vi "Find_Slave_Data.vi"(4 "Process data parameters in":T2={"Stop loop"={"Settings changed?"=FALSE, "Stop?"=refnum}, "Button refs"={"Stop program"=refnum, "Save settings"=refnum, "DAQ mode"=refnum, "Reset settings"=refnum, "Apply settings"=refnum, "Reset MAS"=refnum, "Reset SLV"=refnum, "Local DBase?"=refnum, "Last value DBase"=FALSE, "Database"=refnum, "Calibration"=refnum, "Save settings 2"=refnum}, "Process messages"={"Process message mode"=enum."Error", "Slave data?"=FALSE, "Length get settings message"=0, "Delta time"=0.0, "Data_Filter"={"Filter_Data"=FALSE, "Use_Thresh"=FALSE, "Reduce data?"=FALSE}, "Time_difference_stack"=[], "Starting sec"=0, "Ending sec"=0, "Ending sec 2"=0, "MAS_Page_Thresh"=refnum, "SLV_Page_Thresh"=refnum, "Database"=refnum}, "Settings state"={"MAS locked?"=refnum, "SLV locked?"=refnum}, "Mode"={"Mode"=enum."Dialog", "Expert?"=FALSE, "Dialog?"=FALSE}, "Alignment parameters"=refnum, "Timer parameters"=refnum, "Files"={"Path config file"=path "", "Path def. ini file"=path "", "Path ini file 1"=path "", "Path ini file 2"=path "", "Path RBF file"=path ""}, "Time difference"=refnum, "Alignment"={"GEN_Page_Calibrate"=refnum, "MAS_Page_Gain"=refnum, "MAS_Page_Offset"=refnum, "SLV_Page_Gain"=refnum, "SLV_Page_Offset"=refnum, "MAS_Page_Common"=refnum, "SLV_Page_Common"=refnum}, "Page Statistics"=refnum}, 6 "Queues":T11, 7 "One Second in":T12[](array[typedef]) {"Ch1 High" format="%0.0f"}, 8 "Status/Errors in":refnum<vi>, 9 "Time master":dbl, 10 "GPS timestamp master":T13, 11 "Devices":T14) -> (0 "Status/Errors out":refnum<vi>, 1 "Time delta slave":dbl, 2 "Slave data":u8[](array[numeric]), 3 "Found SLV data?":T1, 5 "One Second out":T12[](array[typedef]) {"Ch1 High" format="%0.0f"})   [LabVIEW 2010]
uses:
  Controls/Devices.ctl
  Controls/GPS_Timestamp.ctl
  Controls/One_Second.ctl
  Controls/Queues.ctl
  Controls/Process_Data_Parameters.ctl
  Controls/Stop_Loop.ctl
  Controls/Button_Refs.ctl
  Controls/Process_Messages.ctl
  Controls/Process_Message_Mode.ctl
  Controls/Settings_State.ctl
  Controls/Mode.ctl
  Controls/Files.ctl
  Controls/Page_Calibration.ctl
  Controls/Found_SLV_Data.ctl
  Controls/Comparison_Result.ctl
  Controls/Master.ctl
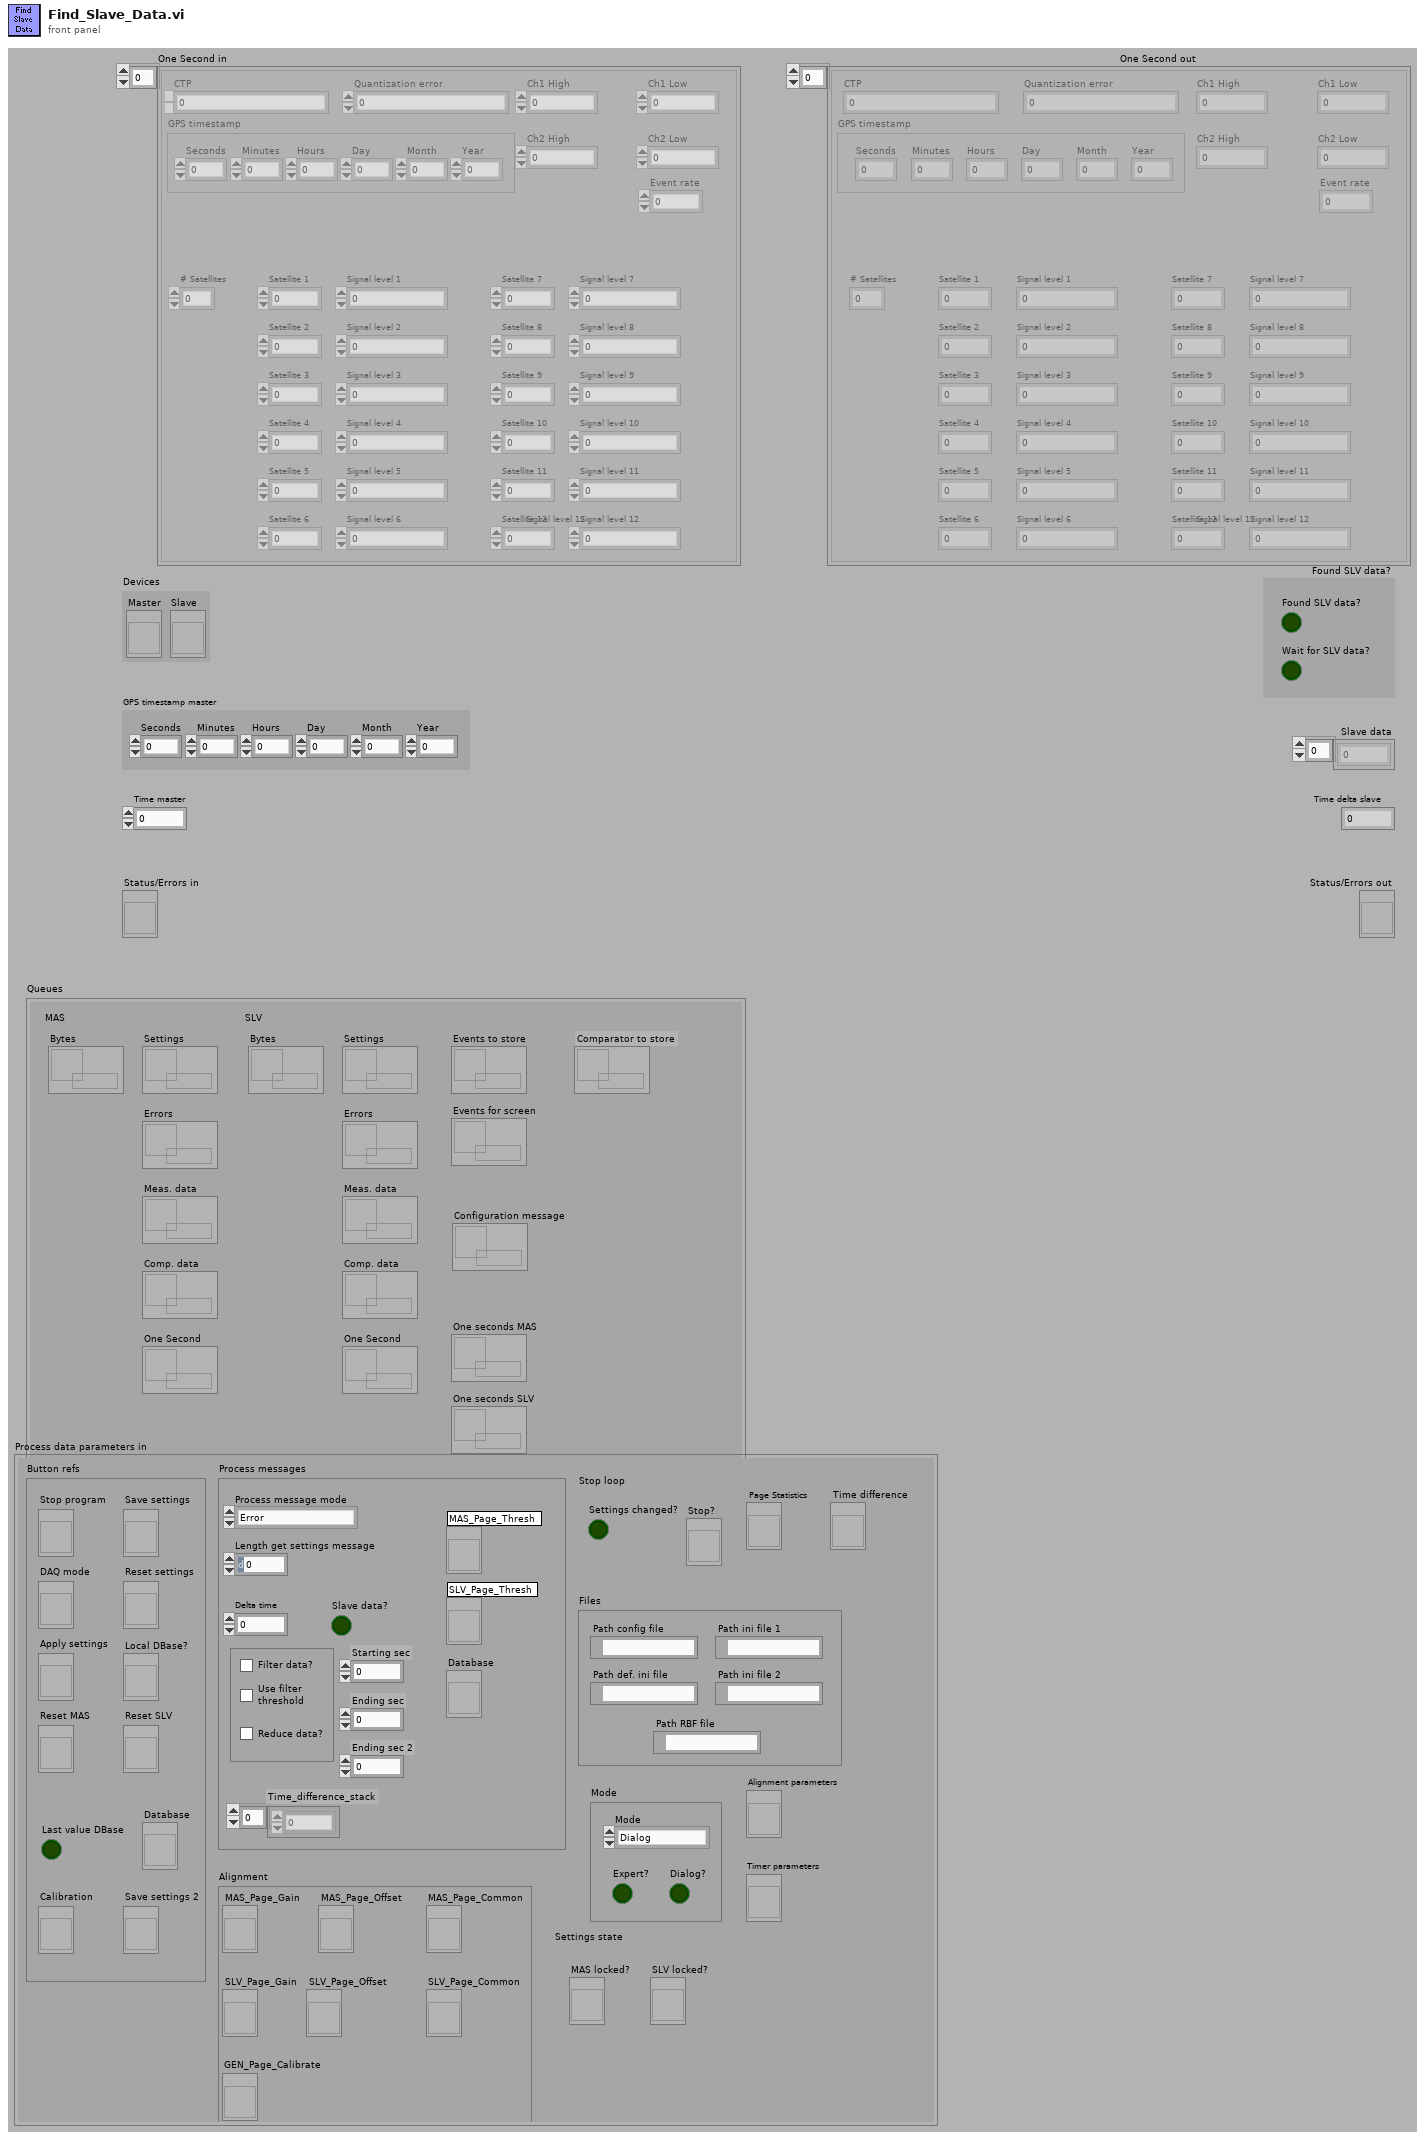
[diagram p1: front panel]
types:
  T1 = typedef "Found_SLV_Data.ctl" = cluster{"Found SLV data?":bool, "Wait for SLV data?":bool}
  T2 = typedef "Process_Data_Parameters.ctl" = cluster{"Stop loop":T3, "Button refs":T4, "Process messages":T5, "Settings state":T7, "Mode":T8, "Alignment parameters":refnum<vi>, "Timer parameters":refnum<vi>, "Files":T9, "Time difference":refnum<vi>, "Alignment":T10, "Page Statistics":refnum<vi>}
  T3 = typedef "Stop_Loop.ctl" = cluster{"Settings changed?":bool, "Stop?":refnum<vi>}
  T4 = typedef "Button_Refs.ctl" = cluster{"Stop program":refnum<vi>, "Save settings":refnum<vi>, "DAQ mode":refnum<vi>, "Reset settings":refnum<vi>, "Apply settings":refnum<vi>, "Reset MAS":refnum<vi>, "Reset SLV":refnum<vi>, "Local DBase?":refnum<vi>, "Last value DBase":bool, "Database":refnum<vi>, "Calibration":refnum<vi>, "Save settings 2":refnum<vi>}
  T5 = typedef "Process_Messages.ctl" = cluster{"Process message mode":T6, "Slave data?":bool, "Length get settings message":i32, "Delta time":dbl, "Data_Filter":cluster{"Filter_Data":bool, "Use_Thresh":bool, "Reduce data?":bool}, "Time_difference_stack":u64[], "Starting sec":u64, "Ending sec":u64, "Ending sec 2":u64, "MAS_Page_Thresh":refnum<vi>, "SLV_Page_Thresh":refnum<vi>, "Database":refnum<vi>}
  T6 = typedef "Process_Message_Mode.ctl" = enum16{"Error", "Measurement data", "Comparator data", "One Second"}
  T7 = typedef "Settings_State.ctl" = cluster{"MAS locked?":refnum<vi>, "SLV locked?":refnum<vi>}
  T8 = typedef "Mode.ctl" = cluster{"Mode":enum8{"Stop", "Dialog", "Hisparc II", "Hisparc II DAQ", "Alignment"}, "Expert?":bool, "Dialog?":bool}
  T9 = typedef "Files.ctl" = cluster{"Path config file":path, "Path def. ini file":path, "Path ini file 1":path, "Path ini file 2":path, "Path RBF file":path}
  T10 = typedef "Page_Calibration.ctl" = cluster{"GEN_Page_Calibrate":refnum<vi>, "MAS_Page_Gain":refnum<vi>, "MAS_Page_Offset":refnum<vi>, "SLV_Page_Gain":refnum<vi>, "SLV_Page_Offset":refnum<vi>, "MAS_Page_Common":refnum<vi>, "SLV_Page_Common":refnum<vi>}
  T11 = typedef "Queues.ctl" = cluster{"MAS":cluster{"Bytes":refnum<queue>, "Settings":refnum<queue>, "Errors":refnum<queue>, "Meas. data":refnum<queue>, "One Second":refnum<queue>, "Comp. data":refnum<queue>}, "SLV":cluster{"Bytes":refnum<queue>, "Settings":refnum<queue>, "Errors":refnum<queue>, "Meas. data":refnum<queue>, "One Second":refnum<queue>, "Comp. data":refnum<queue>}, "Events to store":refnum<queue>, "Events for screen":refnum<queue>, "One seconds MAS":refnum<queue>, "One seconds SLV":refnum<queue>, "Configuration message":refnum<queue>, "Comparator to store":refnum<queue>}
  T12 = typedef "One_Second.ctl" = cluster{"GPS timestamp":T13, "CTP":u32, "Quantization error":u32, "Ch1 High":u16, "Ch1 Low":u16, "Ch2 High":u16, "Ch2 Low":u16, "Event rate":u16, "# Satellites":u8, "Satellite 1":u8, "Satellite 2":u8, "Satellite 3":u8, "Satellite 4":u8, "Satellite 5":u8, "Satellite 6":u8, "Signal level 1":sgl, "Signal level 2":sgl, "Signal level 3":sgl, "Signal level 4":sgl, "Signal level 5":sgl, "Signal level 6":sgl, "Satellite 7":u8, "Satellite 8":u8, "Satellite 9":u8, "Satellite 10":u8, "Satellite 11":u8, "Satellite 12":u8, "Signal level 7":sgl, "Signal level 8":sgl, "Signal level 9":sgl, "Signal level 10":sgl, "Signal level 11":sgl, "Signal level 12":sgl}
  T13 = typedef "GPS_Timestamp.ctl" = cluster{"Seconds":u8, "Minutes":u8, "Hours":u8, "Day":u8, "Month":u8, "Year":u16}
  T14 = typedef "Devices.ctl" = cluster{"Master":refnum<vi>, "Slave":refnum<vi>}
  T15 = typedef "Master.ctl" = enum16{"Master", "Slave", "General"}
  T16 = typedef "Comparison_Result.ctl" = enum16{"equal", "1 < 2", "1 > 2", "error in 1", "error in 2", "error in both"}
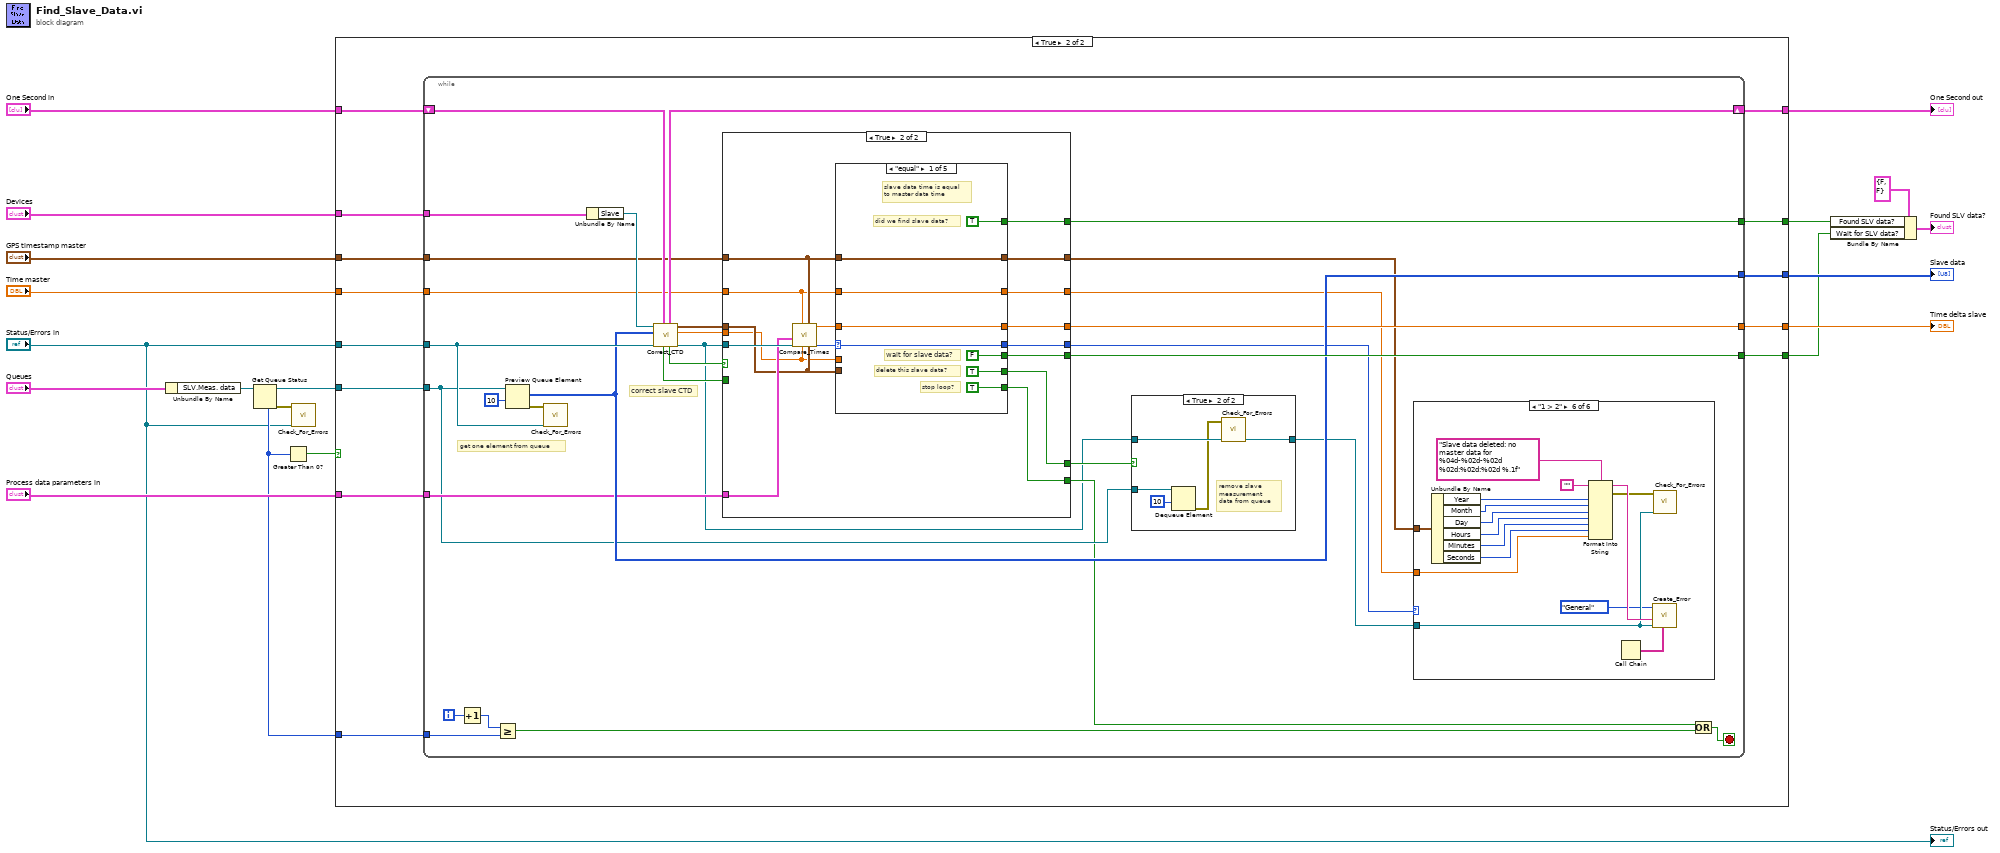
[diagram p0: block diagram]
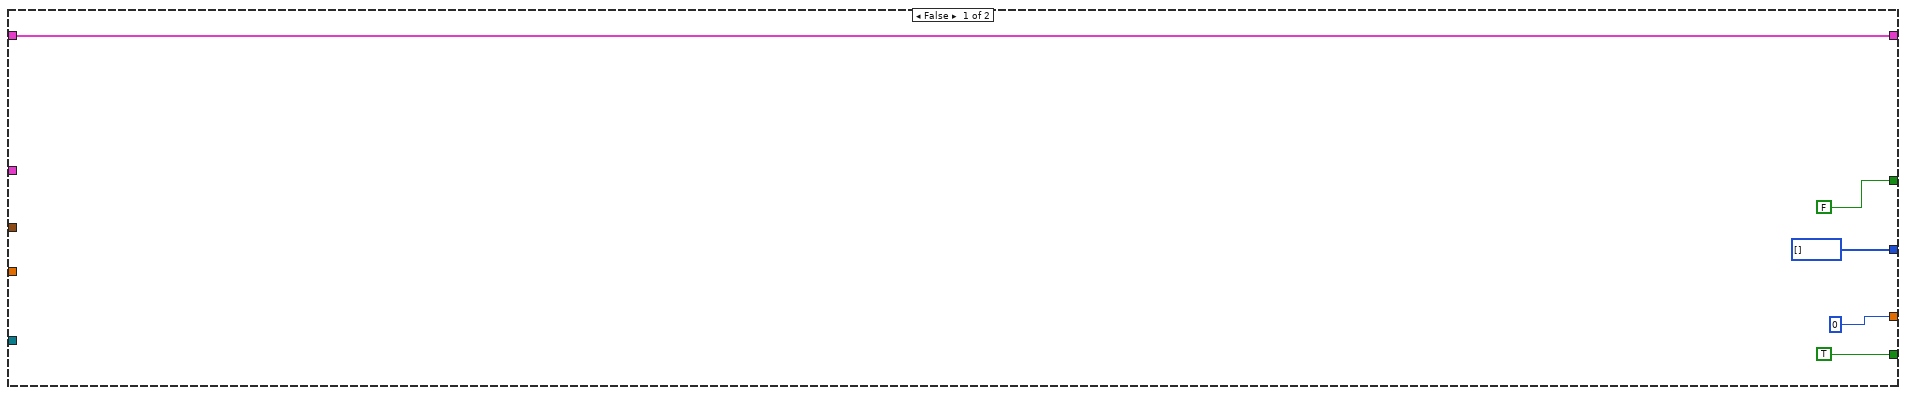
[diagram p2: hidden frame]
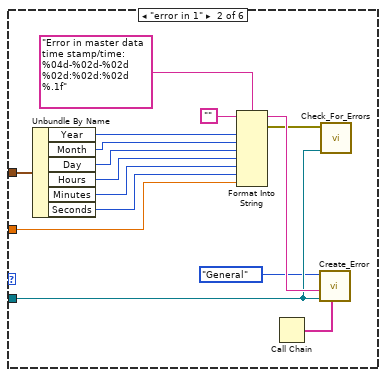
[diagram p4: hidden frame]
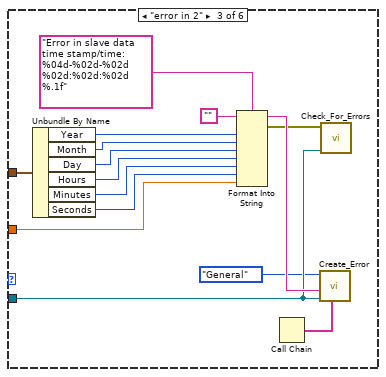
[diagram p5: hidden frame]
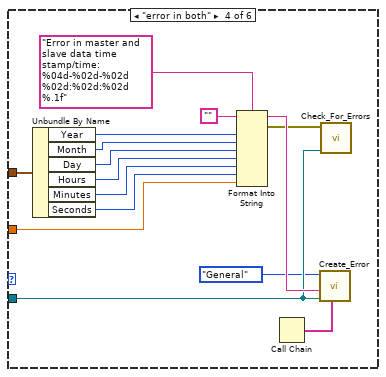
[diagram p6: hidden frame]
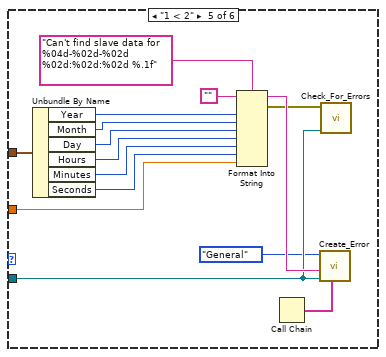
[diagram p7: hidden frame]
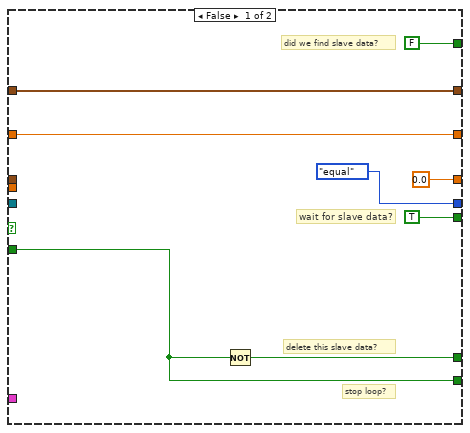
[diagram p9: hidden frame]
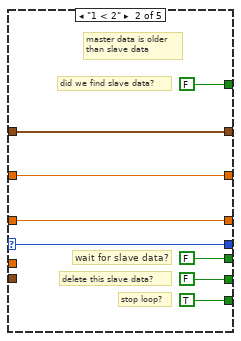
[diagram p10: hidden frame]
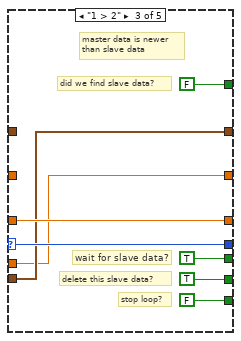
[diagram p11: hidden frame]
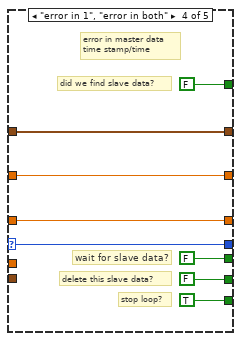
[diagram p12: hidden frame]
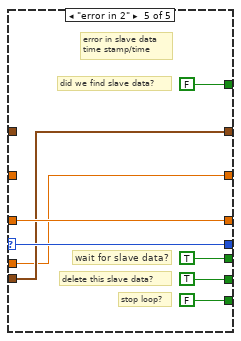
[diagram p13: hidden frame]
diagram:
  n1 = Unbundle By Name("Queues") -> ("SLV.Meas. data"=w12:refnum<queue>)
  n2 = Get Queue Status(queue=w12) -> (queue out=w11:refnum<queue>, error out=w10:errorcluster, # elements in queue=w6:i32)  [unwired: 1 in, 6 out]
  n3 = Greater Than 0?(x=w6) -> (x > 0?=w9:bool)
  n4 = call "Check_For_Errors.vi"("Status/Errors in"="Status/Errors in", "error in"=w10) -> ()  [unwired: 10 out]
  n5 = case shown="True" w9 {
    tunnel: "One Second in" -> [w22 w37]
    tunnel: [w22 w36] -> w18
    tunnel: "Status/Errors in" -> [_ w35]
    tunnel: [FALSE w30] -> w3
    tunnel: [TRUE w31] -> w2
    tunnel: "Devices" -> [_ w34]
    tunnel: "Process data parameters in" -> [_ w33]
    tunnel: "GPS timestamp master" -> [_ w26]
    tunnel: "Time master" -> [_ w25]
    tunnel: w11 -> [_ w32]
    tunnel: [u8[] [] ("Slave data") w29] -> w8
    tunnel: [0 ("CTDM slave") w28] -> w7
    tunnel: w6 -> [_ w27]
    frame False {
    }
    frame True {
      n6 = while {
        tunnel: w35 -> [w65]
        tunnel: w34 -> [w64]
        tunnel: w33 -> [w54]
        tunnel: w26 -> [w53]
        tunnel: w25 -> [w52]
        tunnel: w32 -> [w47]
        tunnel: [w58] -> w31
        tunnel: [w57] -> w30
        tunnel: [w56] -> w29
        tunnel: [w55] -> w28
        tunnel: w27 -> [w50]
        shift-right: [w62] -> w36
        shift-left: w37 -> [w63]
        i -> [w51]
        stop <- w61 stop-if-true
        # "correct slave CTD"
        # "get one element from queue"
        n7 = Increment(x=w51) -> (x+1=w49:i32)
        n8 = Greater Or Equal?(x=w49, y=w50) -> (x >= y?=w48:bool)
        n9 = Preview Queue Element(queue=w47, timeout in ms (-1)=10) -> (element=w56:u8[], error out=w67:errorcluster)  [unwired: 1 in, 2 out]
        n10 = call "Check_For_Errors.vi"("Status/Errors in"=w65, "error in"=w67) -> ()  [unwired: 10 out]
        n11 = Unbundle By Name(w64) -> ("Slave"=w66:refnum<vi>)
        n12 = call "Correct_CTD.vi"("One Second in"=w63, "Status/Errors in"=w65, "Message in"=w56, "Device in"=w66) -> ("Status/Errors out"=w42:refnum<vi>, "Time"=w43:dbl, "GPS timestamp out"=w44:T13, "CTD corrected?"=w60:bool, "One Second out"=w62:T12[], "Wait for tick count?"=w59:bool)  [unwired: 2 out]
        n13 = case shown="True" w60 {
          tunnel: w59 -> [w153 _]
          tunnel: [TRUE ("Wait for tick count?") w171] -> w58
          tunnel: [FALSE w172] -> w57
          tunnel: [0.0 ("CTDM slave") w173] -> w55
          tunnel: w54 -> [_ w166]
          tunnel: w53 -> [w151 w163]
          tunnel: w52 -> [w150 w161]
          tunnel: w44 -> [_ w160]
          tunnel: w43 -> [_ w159]
          tunnel: [w155 w170] -> w46
          tunnel: [w153 w169] -> w45
          tunnel: [Comparison_Result."equal" ("Comparison result") w168] -> w41
          tunnel: w42 -> [_ w167]
          tunnel: [w151 w164] -> w39
          tunnel: [w150 w162] -> w38
          frame False {
            # "stop loop?"
            # "delete this slave data?"
            # "wait for slave data?"
            # "did we find slave data?"
            n14 = Not(x=w153) -> (.not. x?=w155:bool)
          }
          frame True {
            n15 = call "Compare_Times.vi"("Time stamp 2"=w160, "Time stamp 1"=w163, "Time 2"=w159, "Time 1"=w161, "Status/Errors in"=w167, "Process data parameters in"=w166) -> ("Comparison result"=w165:T16, "Time 2 - 1"=w158:dbl)  [unwired: 1 in, 3 out]
            n16 = case shown="\"equal\"" w165 {
              selector: w165 -> [w176 w184 w192 w200 w208]
              tunnel: [w181 w189 w197 w205 w213] -> w173
              tunnel: w158 -> [w181 w189 w197 w205 w213]
              tunnel: [TRUE FALSE FALSE FALSE FALSE] -> w172
              tunnel: [FALSE FALSE TRUE FALSE TRUE] -> w171
              tunnel: [TRUE FALSE TRUE FALSE TRUE] -> w170
              tunnel: [TRUE TRUE FALSE TRUE FALSE] -> w169
              tunnel: [w176 w184 w192 w200 w208] -> w168
              tunnel: [w175 w183 w191 w199 w207] -> w164
              tunnel: w163 -> [w175 w183 _ w199 _]
              tunnel: [w174 w182 w190 w198 w206] -> w162
              tunnel: w161 -> [w174 w182 _ w198 _]
              tunnel: w160 -> [_ _ w191 _ w207]
              tunnel: w159 -> [_ _ w190 _ w206]
              frame "equal" {
                # "slave data time is equal\nto master data time"
                # "stop loop?"
                # "delete this slave data?"
                # "wait for slave data?"
                # "did we find slave data?"
              }
              frame "1 < 2" {
                # "master data is older\nthan slave data"
                # "stop loop?"
                # "delete this slave data?"
                # "wait for slave data?"
                # "did we find slave data?"
              }
              frame "1 > 2" {
                # "master data is newer\nthan slave data"
                # "stop loop?"
                # "delete this slave data?"
                # "wait for slave data?"
                # "did we find slave data?"
              }
              frame "error in 1", "error in both" {
                # "error in master data\ntime stamp/time"
                # "stop loop?"
                # "delete this slave data?"
                # "wait for slave data?"
                # "did we find slave data?"
              }
              frame "error in 2" {
                # "error in slave data\ntime stamp/time"
                # "stop loop?"
                # "delete this slave data?"
                # "wait for slave data?"
                # "did we find slave data?"
              }
            }
          }
        }
        n17 = case shown="True" w46 {
          tunnel: w47 -> [_ w149]
          tunnel: w42 -> [w144 w148]
          tunnel: [w144 w145] -> w40
          frame False {
            # "keep slave measurement\ndata in queue for now"
          }
          frame True {
            # "remove slave\nmeasurement\ndata from queue"
            n18 = Dequeue Element(queue=w149, timeout in ms (-1)=10) -> (error out=w147:errorcluster)  [unwired: 1 in, 3 out]
            n19 = call "Check_For_Errors.vi"("Status/Errors in"=w148, "error in"=w147) -> ("Status/Errors out"=w145:refnum<vi>)  [unwired: 9 out]
          }
        }
        n20 = case shown="\"1 > 2\"" w41 {
          tunnel: w40 -> [_ w72 w87 w102 w117 w132]
          tunnel: w39 -> [_ w82 w97 w112 w127 w142]
          tunnel: w38 -> [_ w70 w85 w100 w115 w130]
          frame Default {
          }
          frame "error in 1" {
            n21 = Unbundle By Name(w82) -> ("Year"=w79:u16, "Month"=w78:u8, "Day"=w77:u8, "Hours"=w76:u8, "Minutes"=w75:u8, "Seconds"=w74:u8)
            n22 = Format Into String(format string="Error in master data time stamp/time: %04d-%02d-%02d %02d:%02d:%02d %.1f", initial string="", w79, w78, w77, w76, w75, w74, w70) -> (resulting string=w73:string, error out=w71:errorcluster)  [unwired: 1 in]
            n23 = Call Chain() -> (call chain=w83:string[])
            n24 = call "Create_Error.vi"("Call chain"=w83, "Status/Errors in"=w72, "HiSPARC error"=w73, "Master?"=Master."General") -> ()  [unwired: 2 in, 6 out]
            n25 = call "Check_For_Errors.vi"("Status/Errors in"=w72, "error in"=w71) -> ()  [unwired: 10 out]
          }
          frame "error in 2" {
            n26 = Unbundle By Name(w97) -> ("Year"=w94:u16, "Month"=w93:u8, "Day"=w92:u8, "Hours"=w91:u8, "Minutes"=w90:u8, "Seconds"=w89:u8)
            n27 = Format Into String(format string="Error in slave data time stamp/time: %04d-%02d-%02d %02d:%02d:%02d %.1f", initial string="", w94, w93, w92, w91, w90, w89, w85) -> (resulting string=w88:string, error out=w86:errorcluster)  [unwired: 1 in]
            n28 = Call Chain() -> (call chain=w98:string[])
            n29 = call "Create_Error.vi"("Call chain"=w98, "Status/Errors in"=w87, "HiSPARC error"=w88, "Master?"=Master."General") -> ()  [unwired: 2 in, 6 out]
            n30 = call "Check_For_Errors.vi"("Status/Errors in"=w87, "error in"=w86) -> ()  [unwired: 10 out]
          }
          frame "error in both" {
            n31 = Unbundle By Name(w112) -> ("Year"=w109:u16, "Month"=w108:u8, "Day"=w107:u8, "Hours"=w106:u8, "Minutes"=w105:u8, "Seconds"=w104:u8)
            n32 = Format Into String(format string="Error in master and slave data time stamp/time: %04d-%02d-%02d %02d:%02d:%02d %.1f", initial string="", w109, w108, w107, w106, w105, w104, w100) -> (resulting string=w103:string, error out=w101:errorcluster)  [unwired: 1 in]
            n33 = Call Chain() -> (call chain=w113:string[])
            n34 = call "Create_Error.vi"("Call chain"=w113, "Status/Errors in"=w102, "HiSPARC error"=w103, "Master?"=Master."General") -> ()  [unwired: 2 in, 6 out]
            n35 = call "Check_For_Errors.vi"("Status/Errors in"=w102, "error in"=w101) -> ()  [unwired: 10 out]
          }
          frame "1 < 2" {
            n36 = Unbundle By Name(w127) -> ("Year"=w124:u16, "Month"=w123:u8, "Day"=w122:u8, "Hours"=w121:u8, "Minutes"=w120:u8, "Seconds"=w119:u8)
            n37 = Format Into String(format string="Can't find slave data for %04d-%02d-%02d %02d:%02d:%02d %.1f", initial string="", w124, w123, w122, w121, w120, w119, w115) -> (resulting string=w118:string, error out=w116:errorcluster)  [unwired: 1 in]
            n38 = Call Chain() -> (call chain=w128:string[])
            n39 = call "Create_Error.vi"("Call chain"=w128, "Status/Errors in"=w117, "HiSPARC error"=w118, "Master?"=Master."General") -> ()  [unwired: 2 in, 6 out]
            n40 = call "Check_For_Errors.vi"("Status/Errors in"=w117, "error in"=w116) -> ()  [unwired: 10 out]
          }
          frame "1 > 2" {
            n41 = Unbundle By Name(w142) -> ("Year"=w139:u16, "Month"=w138:u8, "Day"=w137:u8, "Hours"=w136:u8, "Minutes"=w135:u8, "Seconds"=w134:u8)
            n42 = Format Into String(format string="Slave data deleted: no master data for %04d-%02d-%02d %02d:%02d:%02d %.1f", initial string="", w139, w138, w137, w136, w135, w134, w130) -> (resulting string=w133:string, error out=w131:errorcluster)  [unwired: 1 in]
            n43 = Call Chain() -> (call chain=w143:string[])
            n44 = call "Create_Error.vi"("Call chain"=w143, "Status/Errors in"=w132, "HiSPARC error"=w133, "Master?"=Master."General") -> ()  [unwired: 2 in, 6 out]
            n45 = call "Check_For_Errors.vi"("Status/Errors in"=w132, "error in"=w131) -> ()  [unwired: 10 out]
          }
        }
        n46 = Or(x=w45, y=w48) -> (x .or. y?=w61:bool)
      }
    }
  }
  "Time delta slave" <- w7
  "Slave data" <- w8
  "One Second out" <- w18
  n47 = Bundle By Name(cluster=T1 {"Found SLV data?"=FALSE, "Wait for SLV data?"=FALSE} ("Found SLV data?"), "Found SLV data?"=w3, "Wait for SLV data?"=w2) -> (→"Found SLV data?":T1)
  "Status/Errors out" <- "Status/Errors in"
